vi "FIP_ImageSave.vi"(9 "File Name":string, 11 "Image":T1) -> ()   [LabVIEW 2023]
uses:
  <vilib>/vision/Image Controls.llb/IMAQ Image.ctl
  <vilib>/Utility/error.llb/DialogType.ctl
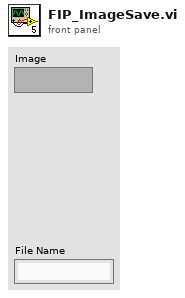
[diagram p1: front panel]
types:
  T1 = typedef "IMAQ Image.ctl" = refnum<image>
  T2 = typedef "DialogType.ctl" = u16
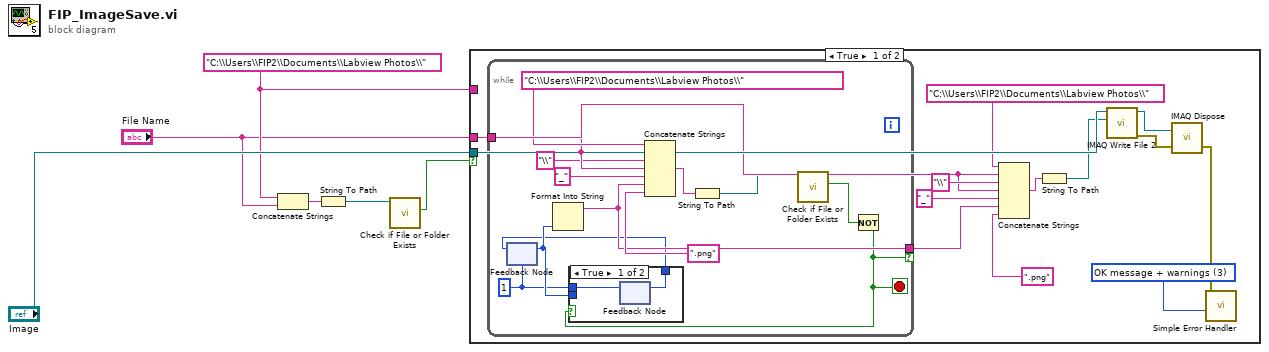
[diagram p0: block diagram]
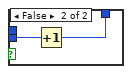
[diagram p2: hidden frame]
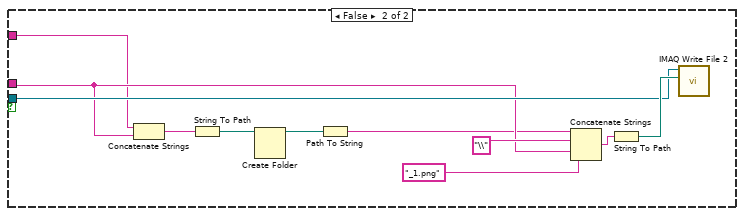
[diagram p3: hidden frame]
diagram:
  w2 = "C:\\Users\\FIP2\\Documents\\Labview Photos\\" ("string")
  n1 = Concatenate Strings(w2, "File Name") -> (w4:string)
  n2 = String To Path(string=w4) -> (path=w3:path)
  n3 = call <vilib>:"Check if File or Folder Exists.vi"("path"=w3) -> ("file or folder exists?"=w5:bool)  [unwired: 8 in, 2 out]
  n4 = case shown="True" w5 {
    tunnel: "Image" -> [w19 w45]
    tunnel: "File Name" -> [w14 w40]
    tunnel: w2 -> [_ w37]
    frame True {
      w10 = T2 3 items=["no dialog", "OK message", "continue or stop message", "OK message + warnings", "continue/stop + warnings"] ("type of dialog (OK msg:1)")
      n5 = while {
        tunnel: w14 -> [w21]
        tunnel: [w27] -> w12 if=w24
        stop <- w24 stop-if-true
        w23 = 1 ("Border Size")
        n6 = feedback #1(w23) -> (w26:i32)
        n7 = Format Into String(w26) -> (resulting string=w27:string)  [unwired: 3 in, 1 out]
        n8 = Concatenate Strings("C:\\Users\\FIP2\\Documents\\Labview Photos\\" ("string"), w21, "\\" ("string"), w21, "_" ("string"), w27, ".png" ("string")) -> (w32:string)
        n9 = String To Path(string=w32) -> (path=w31:path)
        n10 = call <vilib>:"Check if File or Folder Exists.vi"("path"=w31) -> ("file or folder exists?"=w30:bool)  [unwired: 8 in, 2 out]
        n11 = Not(x=w30) -> (.not. x?=w24:bool)
        n12 = case shown="True" w24 {
          tunnel: w26 -> [_ w36]
          tunnel: [w33 w35] -> w25
          tunnel: w23 -> [w34 _]
          frame True {
            n13 = feedback #2() -> (w33:i32)  [unwired: 1 in]
            n14 = feedback-in #2(w34) -> ()
          }
          frame False {
            n15 = Increment(x=w36) -> (x+1=w35:i32)
          }
        }
        n16 = feedback-in #1(w25) -> ()
      }
      n17 = Concatenate Strings("C:\\Users\\FIP2\\Documents\\Labview Photos\\" ("string"), w14, "\\" ("string"), w14, "_" ("string"), w12, ".png" ("string")) -> (w17:string)
      n18 = String To Path(string=w17) -> (path=w16:path)
      n19 = call-poly "IMAQ Write File 2"("File Path"=w16, "Image"=w19) -> ("error out"=w7:errorcluster, "Image Out (duplicate)"=w8:T1)  [unwired: 8 in]
      n20 = call "IMAQ Dispose"("Image"=w8, "error in (no error)"=w7) -> ("error out"=w9:errorcluster)  [unwired: 4 in]
      n21 = call <vilib>:"Simple Error Handler.vi"("type of dialog (OK msg:1)"=w10, "error in (no error)"=w9) -> ()  [unwired: 8 out]
    }
    frame False {
      n22 = Concatenate Strings(w37, w40) -> (w41:string)
      n23 = String To Path(string=w41) -> (path=w42:path)
      n24 = Create Folder(path (use dialog)=w42) -> (created path=w39:path)  [unwired: 2 in, 2 out]
      n25 = Path To String(path=w39) -> (string=w38:string)
      n26 = Concatenate Strings(w38, "\\" ("string"), w40, "_1.png" ("string")) -> (w47:string)
      n27 = String To Path(string=w47) -> (path=w46:path)
      n28 = call-poly "IMAQ Write File 2"("File Path"=w46, "Image"=w45) -> ()  [unwired: 8 in, 2 out]
    }
  }
